vi "Tab Control - Get Tab Control Ref By Name.vi"(8 "error in (no error)":errorcluster, 10 "control label":string, 11 "page ref":refnum<vi>) -> (0 "error out":errorcluster, 3 "control ref out":refnum<vi>)   [LabVIEW 2020]
doc: "Gets page control item ref by its name."
uses:
  <vilib>/Utility/error.llb/Error Cluster From Error Code.vi
  <vilib>/ErrorRing/Error Ring.xnode
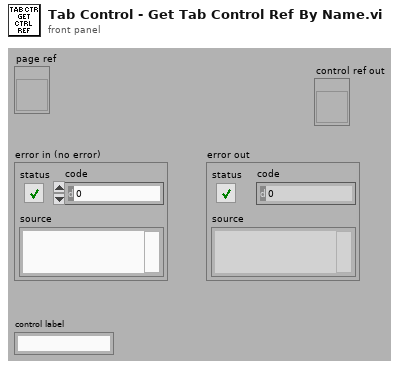
[diagram p1: front panel]
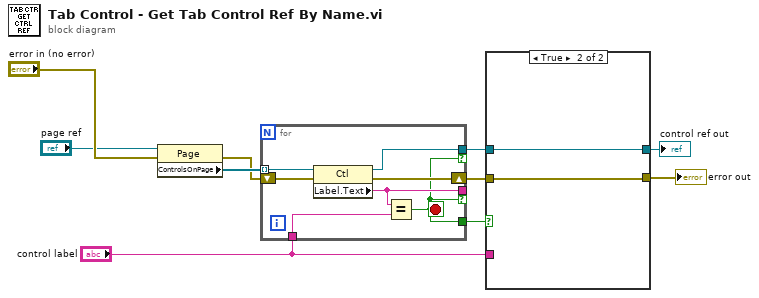
[diagram p0: block diagram]
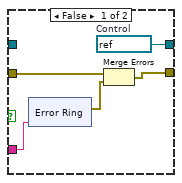
[diagram p2: hidden frame]
diagram:
  n1 = property class="Page"(reference="page ref", error in="error in (no error)") -> (error out=w6:errorcluster, "ControlsOnPage"=w7:refnum<vi>[])  [unwired: 1 out]
  n2 = for {
    tunnel: w7 -> [w17] mode=indexing
    tunnel: [w15] -> _ if=w11
    tunnel: [w11] -> w5
    shift-right: [w14] -> w4
    shift-left: w6 -> [w16]
    tunnel: "control label" -> [w13]
    tunnel: [w12] -> w3 if=w11
    stop <- w11 stop-if-true
    n3 = property class="Ctl"(reference=w17, error in=w16) -> (reference out=w12:refnum<vi>, error out=w14:errorcluster, "Label.Text"=w15:string)
    n4 = Equal?(x=w15, y=w13) -> (x = y?=w11:bool)
  }
  n5 = case shown="True" w5 {
    tunnel: w4 -> [w22 w31]
    tunnel: [w20 w31] -> w10
    tunnel: [w18 w30] -> w1
    tunnel: w3 -> [_ w30]
    tunnel: "control label" -> [w19 _]
    frame False {
      w18 = refnum<vi> refnum  # Control
      n6 = xnode "Error Ring"("parameter 0"=w19) -> ("error out"=w21:errorcluster)
      n7 = Merge Errors(w22, w21) -> (w20:errorcluster)
    }
    frame True {
    }
  }
  "error out" <- w10
  "control ref out" <- w1
